vi "Day06-02_샘플 수집_거리 측정.vi"() -> ()   [LabVIEW 2021]
uses:
  <vilib>/DAQmx/read.llb/DAQmx Read (Analog Wfm 1Chan NSamp).vi
  <vilib>/DAQmx/create/channels.llb/DAQmx Create Channel (AI-Voltage-Basic).vi
  <vilib>/DAQmx/configure/timing.llb/DAQmx Timing (Sample Clock).vi
  <vilib>/DAQmx/miscellaneous.llb/DAQmx Fill In Error Info.vi
  <vilib>/DAQmx/read.llb/DAQmx Read (Analog DBL 1Chan 1Samp).vi
panel:
  in  "정지 3":bool
  out "x-y 2":u32
  out "웨이브폼 차트 2":waveform(dbl)(graph)
  out "웨이브폼 차트":waveform(dbl)(graph)
  out "x-y":u32
  in  "정지 2":bool
  out "웨이브폼 차트":waveform(dbl)(graph)
  out "웨이브폼 차트":dbl(graph)
  in  "정지":bool
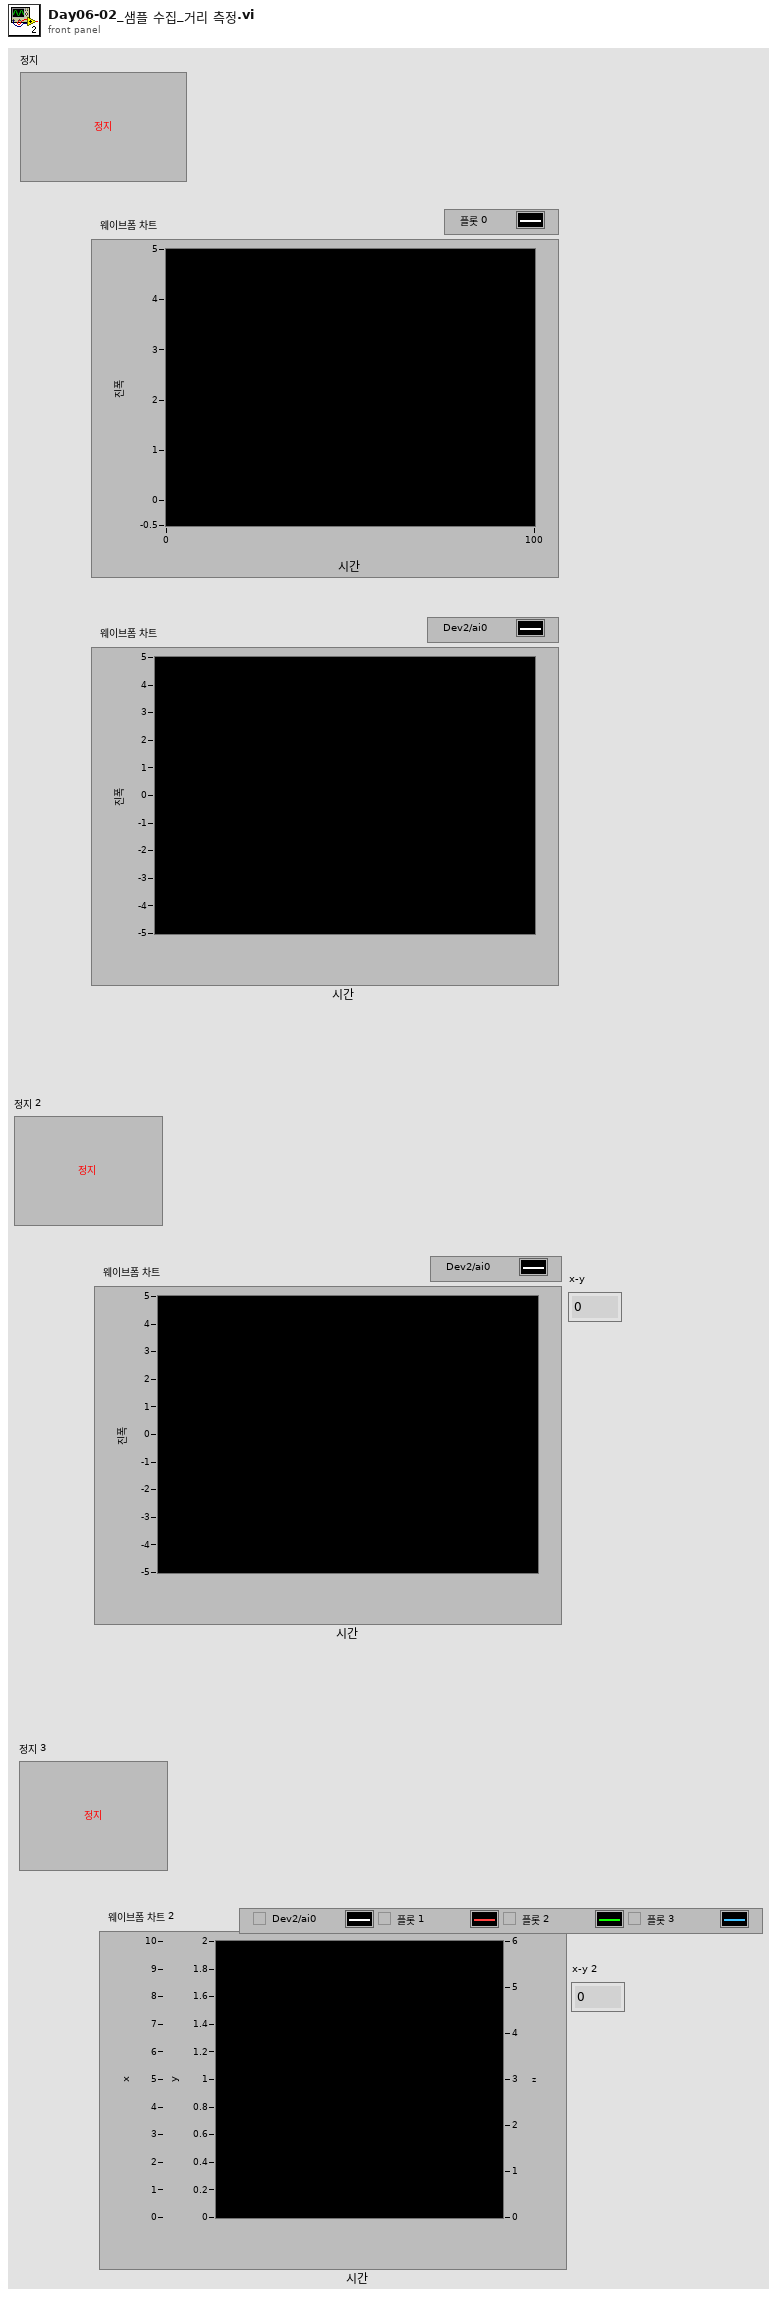
[diagram p1: front panel]
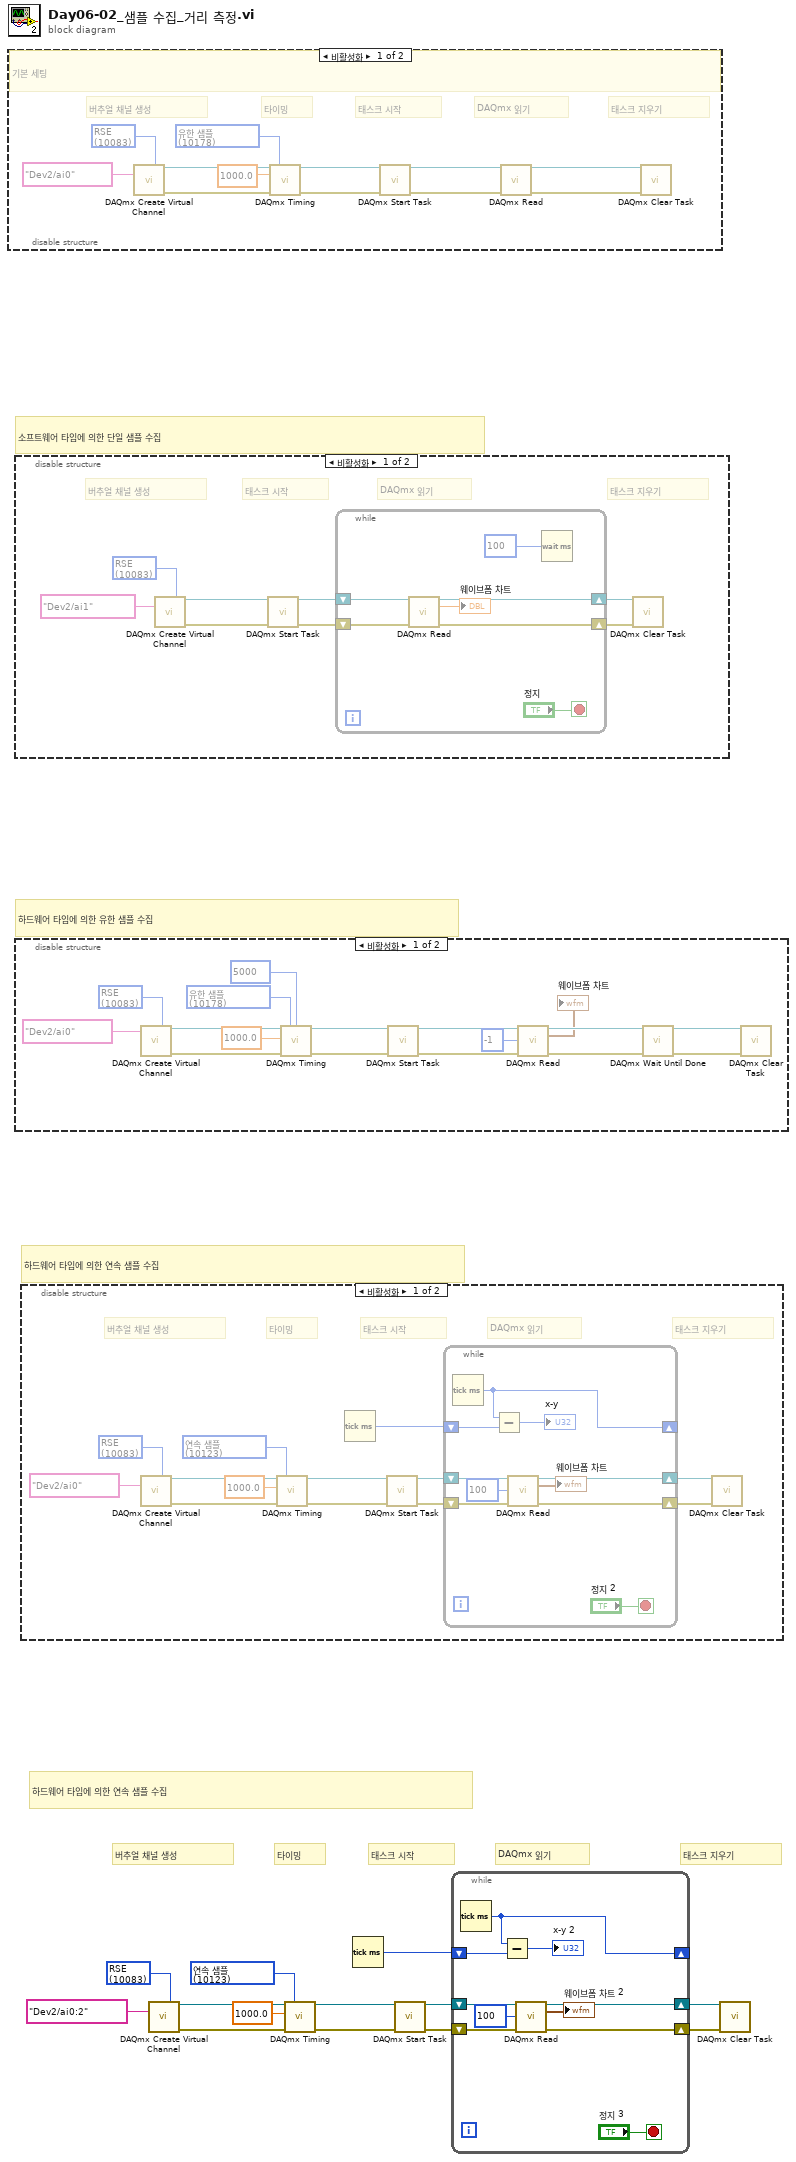
[diagram p0: block diagram]
diagram:
  w3 = 10123 items=["유한 샘플"=10178, "연속 샘플"=10123, "하드웨어 타이밍에 의한 단일 포인트"=12522] ("sample mode")
  w5 = 10083 items=["기본"=-1, "RSE"=10083, "NRSE"=10078, "차동"=10106, "유사 차동"=12529] ("input terminal configuration")
  # "타이밍"
  # "태스크 지우기"
  # "DAQmx 읽기"
  # "태스크 시작"
  # "버추얼 채널 생성"
  # "하드웨어 타임에 의한 연속 샘플 수집"
  # "하드웨어 타임에 의한 연속 샘플 수집"
  # "하드웨어 타임에 의한 유한 샘플 수집"
  # "소프트웨어 타임에 의한 단일 샘플 수집"
  n1 = disable-structure shown="비활성화" {
    frame Disabled {
      w15 = 10178 items=["유한 샘플"=10178, "연속 샘플"=10123, "하드웨어 타이밍에 의한 단일 포인트"=12522] ("sample mode")
      w16 = 10083 items=["기본"=-1, "RSE"=10083, "NRSE"=10078, "차동"=10106, "유사 차동"=12529] ("input terminal configuration")
      # "타이밍"
      # "태스크 지우기"
      # "DAQmx 읽기"
      # "태스크 시작"
      # "버추얼 채널 생성"
      # "기본 세팅"
      n2 = call-poly <vilib>:"DAQmx Create Virtual Channel.vi"("input terminal configuration"=w16, "physical channels"=tag "Dev2/ai0") -> ("task out"=w25:refnum<k21>, "error out"=w24:errorcluster)  [unwired: 12 in]
      n3 = call-poly <vilib>:"DAQmx Timing.vi"("task/channels in"=w25, "sample mode"=w15, "rate"=1000.0, "error in"=w24) -> ("task out"=w23:refnum<k21>, "error out"=w22:errorcluster)  [unwired: 10 in]
      n4 = call <vilib>:"DAQmx Start Task.vi"("task/channels in"=w23, "error in"=w22) -> ("task out"=w20:refnum<k21>, "error out"=w19:errorcluster)  [unwired: 12 in]
      n5 = call-poly <vilib>:"DAQmx Read.vi"("task/channels in"=w20, "error in"=w19) -> ("task out"=w18:refnum<k21>, "error out"=w17:errorcluster)  [unwired: 11 in, 1 out]
      n6 = call <vilib>:"DAQmx Clear Task.vi"("task in"=w18, "error in"=w17) -> ()  [unwired: 13 in, 1 out]
    }
    frame Enabled {
    }
  }
  n7 = disable-structure shown="비활성화" {
    frame Disabled {
      w26 = 10083 items=["기본"=-1, "RSE"=10083, "NRSE"=10078, "차동"=10106, "유사 차동"=12529] ("input terminal configuration")
      # "태스크 지우기"
      # "DAQmx 읽기"
      # "태스크 시작"
      # "버추얼 채널 생성"
      n8 = call-poly <vilib>:"DAQmx Create Virtual Channel.vi"("input terminal configuration"=w26, "physical channels"=tag "Dev2/ai1") -> ("task out"=w33:refnum<k21>, "error out"=w32:errorcluster)  [unwired: 12 in]
      n9 = call <vilib>:"DAQmx Start Task.vi"("task/channels in"=w33, "error in"=w32) -> ("task out"=w31:refnum<k21>, "error out"=w30:errorcluster)  [unwired: 12 in]
      n10 = while {
        shift-right: [w38] -> w29
        shift-left: w31 -> [w40]
        shift-right: [w37] -> w28
        shift-left: w30 -> [w39]
        stop <- "정지" stop-if-true
        n11 = call-poly <vilib>:"DAQmx Read.vi"("task/channels in"=w40, "error in"=w39) -> ("task out"=w38:refnum<k21>, "data"=→"웨이브폼 차트":dbl, "error out"=w37:errorcluster)  [unwired: 11 in]
        n12 = Wait (ms)(milliseconds to wait=u32 100 ("대기 시간 (ms)")) -> ()  [unwired: 1 out]
      }
      n13 = call <vilib>:"DAQmx Clear Task.vi"("task in"=w29, "error in"=w28) -> ()  [unwired: 13 in, 1 out]
    }
    frame Enabled {
    }
  }
  n14 = disable-structure shown="비활성화" {
    frame Disabled {
      w45 = 10178 items=["유한 샘플"=10178, "연속 샘플"=10123, "하드웨어 타이밍에 의한 단일 포인트"=12522] ("sample mode")
      w46 = 10083 items=["기본"=-1, "RSE"=10083, "NRSE"=10078, "차동"=10106, "유사 차동"=12529] ("input terminal configuration")
      n15 = call-poly <vilib>:"DAQmx Create Virtual Channel.vi"("input terminal configuration"=w46, "physical channels"=tag "Dev2/ai0") -> ("task out"=w57:refnum<k21>, "error out"=w56:errorcluster)  [unwired: 12 in]
      n16 = call-poly <vilib>:"DAQmx Timing.vi"("task/channels in"=w57, "sample mode"=w45, "samples per channel"=5000, "rate"=1000.0, "error in"=w56) -> ("task out"=w55:refnum<k21>, "error out"=w54:errorcluster)  [unwired: 9 in]
      n17 = call <vilib>:"DAQmx Start Task.vi"("task/channels in"=w55, "error in"=w54) -> ("task out"=w53:refnum<k21>, "error out"=w52:errorcluster)  [unwired: 12 in]
      n18 = call-poly <vilib>:"DAQmx Read.vi"("task/channels in"=w53, "number of samples per channel"=-1, "error in"=w52) -> ("task out"=w51:refnum<k21>, "data"=→"웨이브폼 차트":waveform(dbl), "error out"=w50:errorcluster)  [unwired: 10 in]
      n19 = call <vilib>:"DAQmx Wait Until Done.vi"("task/channels in"=w51, "error in"=w50) -> ("task out"=w49:refnum<k21>, "error out"=w48:errorcluster)  [unwired: 12 in]
      n20 = call <vilib>:"DAQmx Clear Task.vi"("task in"=w49, "error in"=w48) -> ()  [unwired: 13 in, 1 out]
    }
    frame Enabled {
    }
  }
  n21 = disable-structure shown="비활성화" {
    frame Disabled {
      w60 = 10123 items=["유한 샘플"=10178, "연속 샘플"=10123, "하드웨어 타이밍에 의한 단일 포인트"=12522] ("sample mode")
      w62 = 10083 items=["기본"=-1, "RSE"=10083, "NRSE"=10078, "차동"=10106, "유사 차동"=12529] ("input terminal configuration")
      # "타이밍"
      # "태스크 지우기"
      # "DAQmx 읽기"
      # "태스크 시작"
      # "버추얼 채널 생성"
      n22 = call-poly <vilib>:"DAQmx Create Virtual Channel.vi"("input terminal configuration"=w62, "physical channels"=tag "Dev2/ai0") -> ("task out"=w70:refnum<k21>, "error out"=w69:errorcluster)  [unwired: 12 in]
      n23 = call-poly <vilib>:"DAQmx Timing.vi"("task/channels in"=w70, "sample mode"=w60, "rate"=1000.0, "error in"=w69) -> ("task out"=w68:refnum<k21>, "error out"=w67:errorcluster)  [unwired: 10 in]
      n24 = Tick Count (ms)() -> (millisecond timer value=w58:u32)
      n25 = call <vilib>:"DAQmx Start Task.vi"("task/channels in"=w68, "error in"=w67) -> ("task out"=w66:refnum<k21>, "error out"=w65:errorcluster)  [unwired: 12 in]
      n26 = while {
        shift-right: [w78] -> w64
        shift-left: w66 -> [w80]
        shift-right: [w77] -> w63
        shift-left: w65 -> [w79]
        shift-right: [w73] -> _
        shift-left: w58 -> [w74]
        stop <- "정지 2" stop-if-true
        n27 = Tick Count (ms)() -> (millisecond timer value=w73:u32)
        n28 = Subtract(x=w73, y=w74) -> (x-y=→"x-y":u32)
        n29 = call-poly <vilib>:"DAQmx Read.vi"("task/channels in"=w80, "number of samples per channel"=100, "error in"=w79) -> ("task out"=w78:refnum<k21>, "data"=→"웨이브폼 차트":waveform(dbl), "error out"=w77:errorcluster)  [unwired: 10 in]
      }
      n30 = call <vilib>:"DAQmx Clear Task.vi"("task in"=w64, "error in"=w63) -> ()  [unwired: 13 in, 1 out]
    }
    frame Enabled {
    }
  }
  n31 = call-poly <vilib>:"DAQmx Create Virtual Channel.vi"("input terminal configuration"=w5, "physical channels"=tag "Dev2/ai0:2") -> ("task out"=w13:refnum<k21>, "error out"=w12:errorcluster)  [unwired: 12 in]
  n32 = call-poly <vilib>:"DAQmx Timing.vi"("task/channels in"=w13, "sample mode"=w3, "rate"=1000.0, "error in"=w12) -> ("task out"=w11:refnum<k21>, "error out"=w10:errorcluster)  [unwired: 10 in]
  n33 = Tick Count (ms)() -> (millisecond timer value=w1:u32)
  n34 = call <vilib>:"DAQmx Start Task.vi"("task/channels in"=w11, "error in"=w10) -> ("task out"=w9:refnum<k21>, "error out"=w8:errorcluster)  [unwired: 12 in]
  n35 = while {
    shift-right: [w88] -> w7
    shift-left: w9 -> [w90]
    shift-right: [w87] -> w6
    shift-left: w8 -> [w89]
    shift-right: [w83] -> _
    shift-left: w1 -> [w84]
    stop <- "정지 3" stop-if-true
    n36 = Tick Count (ms)() -> (millisecond timer value=w83:u32)
    n37 = Subtract(x=w83, y=w84) -> (x-y=→"x-y 2":u32)
    n38 = call-poly <vilib>:"DAQmx Read.vi"("task/channels in"=w90, "number of samples per channel"=100, "error in"=w89) -> ("task out"=w88:refnum<k21>, "data"=→"웨이브폼 차트 2":waveform(dbl), "error out"=w87:errorcluster)  [unwired: 10 in]
  }
  n39 = call <vilib>:"DAQmx Clear Task.vi"("task in"=w7, "error in"=w6) -> ()  [unwired: 13 in, 1 out]
